vi "SIM Check Error.vi"(7 "min float":dbl, 8 "estimated error":dbl[](array[numeric]), 9 "absolute tolerance":dbl, 10 "relative tolerance":dbl, 11 "Solution":dbl[](array[numeric])) -> (0 "within acceptable err?":bool, 2 "acceptable err/estimated err":dbl, 3 "Solution Out":dbl[](array[numeric]))   [LabVIEW 2014]
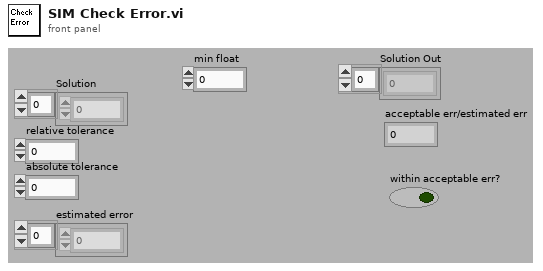
[diagram p1: front panel]
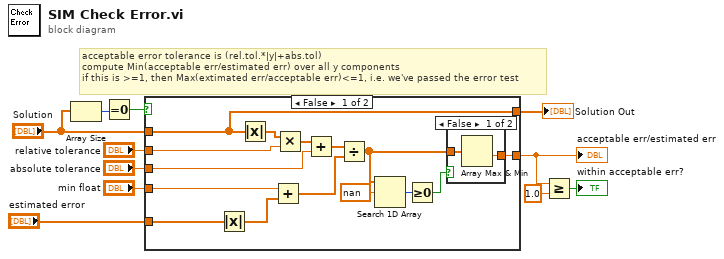
[diagram p0: block diagram]
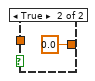
[diagram p2: hidden frame]
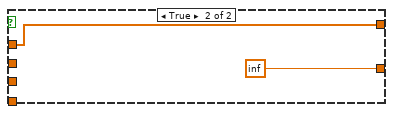
[diagram p3: hidden frame]
diagram:
  # "acceptable error tolerance is (rel.tol.*|y|+abs.tol)\ncompute Min(acceptable err/estimated err) over all y components\nif this is >=1, then Max(extimated err/acceptable err)<=1, i.e. we've passed the error test"
  n1 = Array Size(array="Solution") -> (size(s)=w9:i32)
  n2 = Equal To 0?(x=w9) -> (x = 0?=w8:bool)
  n3 = case shown="False" w8 {
    tunnel: [w26 inf] -> w6
    tunnel: "estimated error" -> [w21 _]
    tunnel: "Solution" -> [w12 w30]
    tunnel: "relative tolerance" -> [w15 _]
    tunnel: "absolute tolerance" -> [w14 _]
    tunnel: "min float" -> [w13 _]
    tunnel: [w12 w30] -> w1
    frame False {
      n4 = Absolute Value(x=w21) -> (abs(x)=w23:dbl[])
      n5 = Absolute Value(x=w12) -> (abs(x)=w24:dbl[])
      n6 = Add(x=w13, y=w23) -> (x+y=w22:dbl[])
      n7 = Multiply(x=w24, y=w15) -> (x*y=w20:dbl[])
      n8 = Add(x=w20, y=w14) -> (x+y=w25:dbl[])
      n9 = Divide(x=w25, y=w22) -> (x/y=w16:dbl[])
      n10 = Search 1D Array(1D array=w16, element=nan) -> (index of element=w18:i32)  [unwired: 1 out]
      n11 = Greater Or Equal To 0?(x=w18) -> (x >= 0?=w17:bool)
      n12 = case shown="False" w17 {
        tunnel: [w28 0.0] -> w26
        tunnel: w16 -> [w27 _]
        frame False {
          n13 = Array Max & Min(array=w27) -> (min value=w28:dbl)  [unwired: 3 out]
        }
        frame True {
        }
      }
    }
    frame True {
    }
  }
  "acceptable err/estimated err" <- w6
  "Solution Out" <- w1
  n14 = Greater Or Equal?(x=w6, y=1.0) -> (x >= y?=→"within acceptable err?":bool)
